vi "Climb Update State.vi"(9 "Stage Finished?":bool, 10 "Current Bar":T1, 11 "Sequence State":T2) -> (2 "Automated Climb State":T3)   [LabVIEW 2020]
uses:
  Implementation/Automated Climb State.ctl
  Implementation/Climb Sequence Stage.ctl
  Implementation/Climb Bar State.ctl
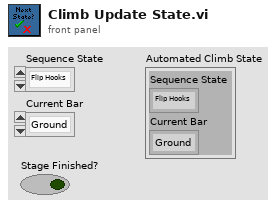
[diagram p1: front panel]
types:
  T1 = typedef "Climb Bar State.ctl" = enum16{"Ground", "Mid", "High", "Traverse"}
  T2 = typedef "Climb Sequence Stage.ctl" = enum16{"Flip Hooks", "Rest on Bar", "Tilt Back", "Tilt To Bar", "Grab Bar", "Pull Up"}
  T3 = typedef "Automated Climb State.ctl" = cluster{"Sequence State":T2, "Current Bar":T1}
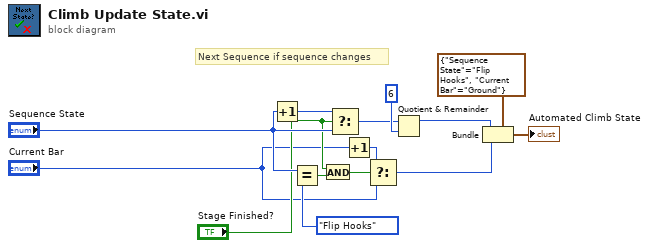
[diagram p0: block diagram]
diagram:
  # "Next Sequence if sequence changes"
  n1 = Increment(x="Sequence State") -> (x+1=w1:T2)
  n2 = Equal?(x="Sequence State", y=Climb_Sequence_Stage."Flip Hooks" ("Sequence State")) -> (x = y?=w11:bool)
  n3 = And(x="Stage Finished?", y=w11) -> (x .and. y?=w2:bool)
  n4 = Select(t=w1, s="Stage Finished?", f="Sequence State") -> (s? t:f=w7:T2)
  n5 = Increment(x="Current Bar") -> (x+1=w4:T1)
  n6 = Select(t=w4, s=w2, f="Current Bar") -> (s? t:f=w3:T1)
  n7 = Quotient & Remainder(x=w7, y=6) -> (x-y*floor(x/y)=w9:i32)  [unwired: 1 out]
  n8 = Bundle(cluster=T3 {"Sequence State"=enum."Flip Hooks", "Current Bar"=enum."Ground"} ("t"), "Sequence State"=w9, "Current Bar"=w3) -> (→"Automated Climb State":T3)
